vi "Variable Setup GUI.vi"(11 "error in (no error)":errorcluster) -> (8 "OK":bool, 15 "error out":errorcluster)   [LabVIEW 2011]
uses:
  Common/Variable List Common Analog.ctl
  Scaling.ctl
  Action List.ctl
  Alarm Responce.ctl
  Limits.ctl
  Alarm Setup.ctl
  User Setting Analog Channel.ctl
  Update frequensies.ctl
panel:
  out "Sampling Rate":T1
  out "Description":string
  out "Unit":string
  out "Name":string
  in  "User Selectable":T2 {"Limits and responces"."Limits"."H" format="%.3f"; "Limits and responces"."Limits"."L" format="%.3f"; "Limits and responces"."Limits"."HH" format="%.3f"; "Limits and responces"."Limits"."LL" format="%.3f"; "Limits and responces"."HH"."Action" items=["No Action", "Turn Off HV"]; "Limits and responces"."H"."Action" items=["No Action", "Turn Off HV"]; "Limits and responces"."L"."Action" items=["No Action", "Turn Off HV"]; "Limits and responces"."LL"."Action" items=["No Action", "Turn Off HV"]; "Limits and responces"."Technical Error"."Action" items=["No Action", "Turn Off HV"]; "Scaling"."Offset" format="%.5f"; "Scaling"."Gain" format="%.5f"}
  in  "List of variables":i32(listbox)
  out "Mode":bool
  in  "Help":bool
  in  "Cancel":bool
  in  "OK":bool
  # "Information"
  # "Tab header s can be changed as wanted\n\nCustom can be used for completly ccutom behavior,\nmust then highjack  an other hidden page, for settings"
  # "Add custom behavior taht cvan not be replicated by a simple cluster with valisdity checking"
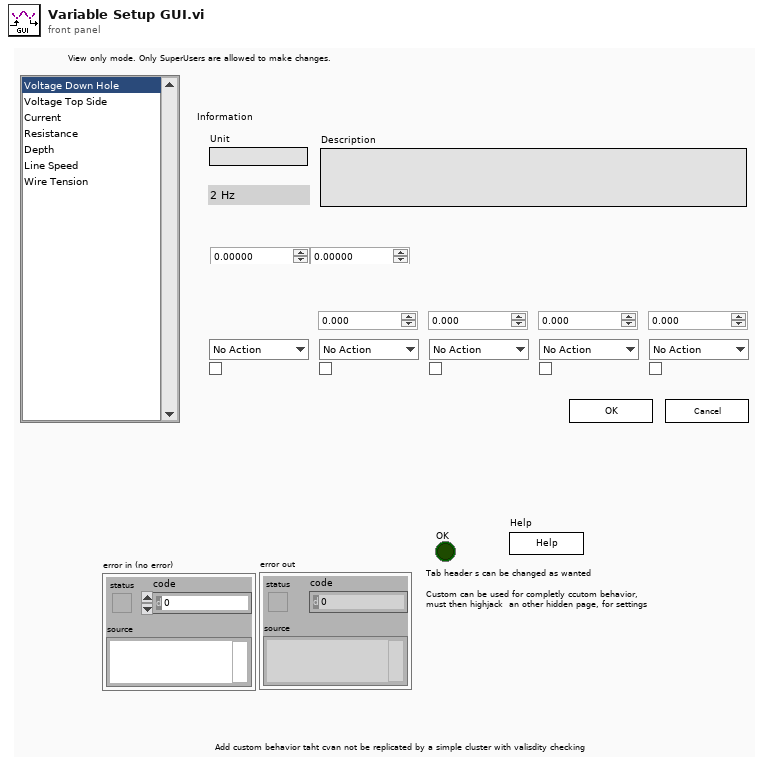
[diagram p1: front panel]
types:
  T1 = typedef "Update frequensies.ctl" = enum16{"2 Hz", "1 Hz", "0.1 Hz"}
  T2 = typedef "User Setting Analog Channel.ctl" = cluster{"Scaling":T3, "Limits and responces":T4}
  T3 = typedef "Scaling.ctl" = cluster{"Gain":dbl, "Offset":dbl}
  T4 = typedef "Alarm Setup.ctl" = cluster{"Technical Error":T5, "LL":T5, "L":T5, "H":T5, "HH":T5, "Limits":T7}
  T5 = typedef "Alarm Responce.ctl" = cluster{"Action":T6, "Alarm":bool}
  T6 = typedef "Action List.ctl" = u16
  T7 = typedef "Limits.ctl" = cluster{"LL":dbl, "L":dbl, "H":dbl, "HH":dbl}
  T8 = enum16{"GET", "SET", "Get from Ini", "Put in Ini"}
  T9 = typedef "User Indikator.ctl" = cluster{"User Name":string, "Super User":T10}
  T10 = typedef "Super User bool indikator.ctl" = bool
  T11 = typedef "Variable List Common Analog.ctl" = enum16{"HVPSU Head Voltage", "HVPSU TS Voltage", "HVPSU Current", "PCP Cable Resistance", "Winch Depth", "Winch Line Speed", "Winch Wire Tension"}
  T12 = enum8{"Enabled", "Disabled", "Disabled and Grayed Out"}
  T13 = typedef "User Setting Analog Channel Bg.ctl" = cluster{"Scaling":T3, "Limits and responces":T14, "Allow Graph selection by user":bool, "Unit":u16}
  T14 = typedef "Alarm Setup Analog.ctl" = cluster{"Technical Error(NA)":T5, "LL":T5, "L":T5, "H":T5, "HH":T5, "Limits":T7}
  T15 = typedef "Fixed Analog Channel Definition.ctl" = cluster{"ID":u16, "Name":string, "Quantity":T16, "Unit":string, "Maximum upd":T1, "Comment":string, "Help file Name":string, "Help file Section ":string, "Category":T17, "User adjustable Scaling":bool, "Default Scaling":T3, "In use":bool, "Default Unit":i32}
  T16 = typedef "Quantity enum.ctl" = enum16{"Acceleration", "Angle", "Current", "Force", "Distance", "Pressure", "Resistance", "Rotational Speed", "Speed", "Temperature", "Tension", "Torque", "Voltage", "Weight"}
  T17 = typedef "Channel catagory Enum.ctl" = enum16{"No Category", "Power", "Temperature", "Pressure"}
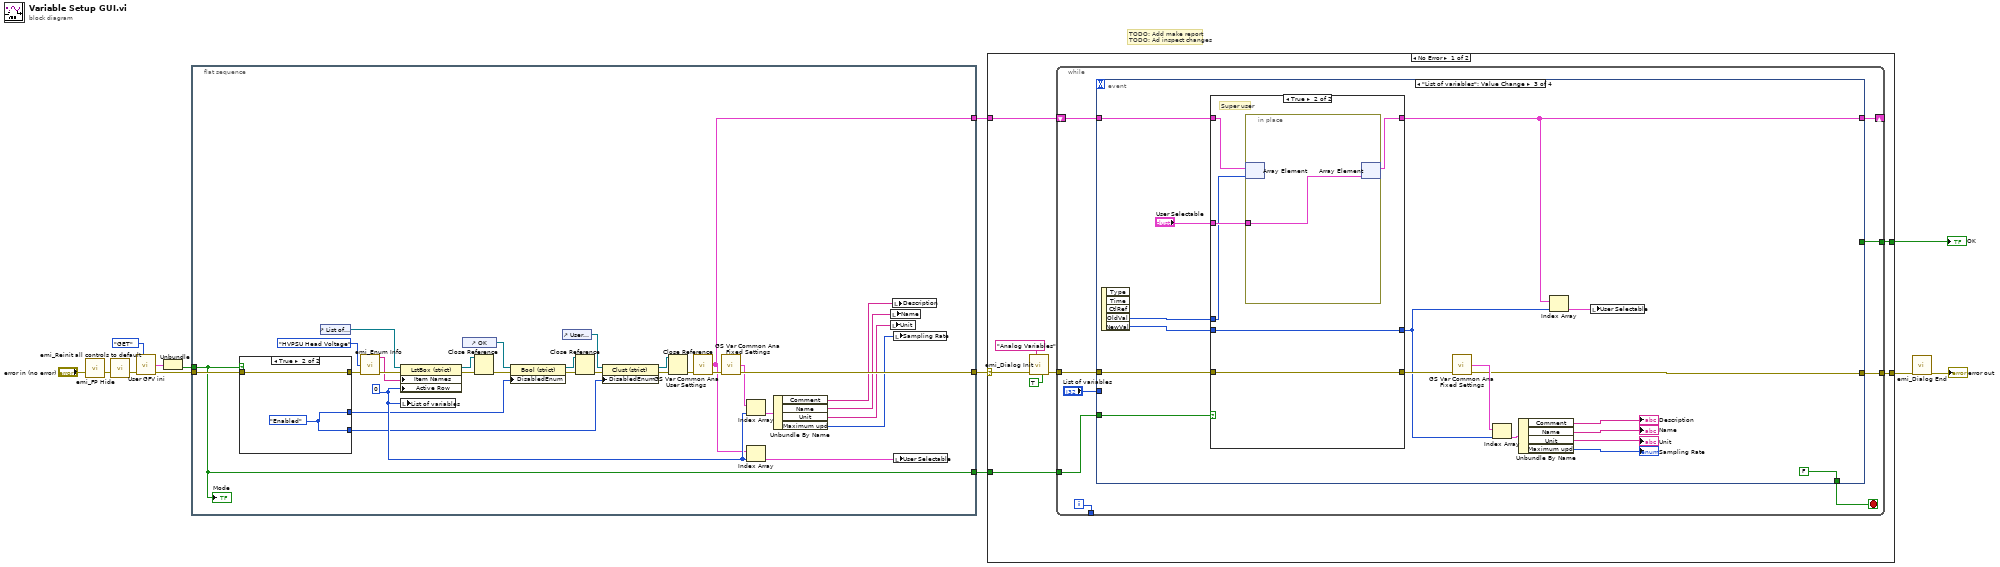
[diagram p0: block diagram]
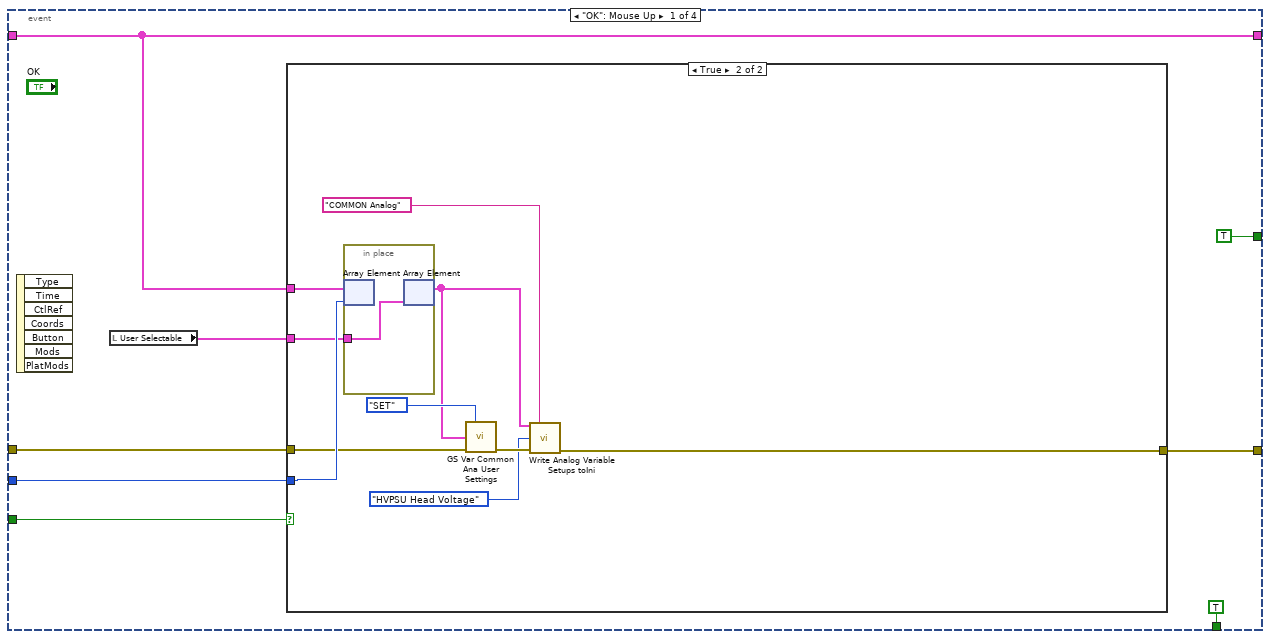
[diagram p2: hidden frame]
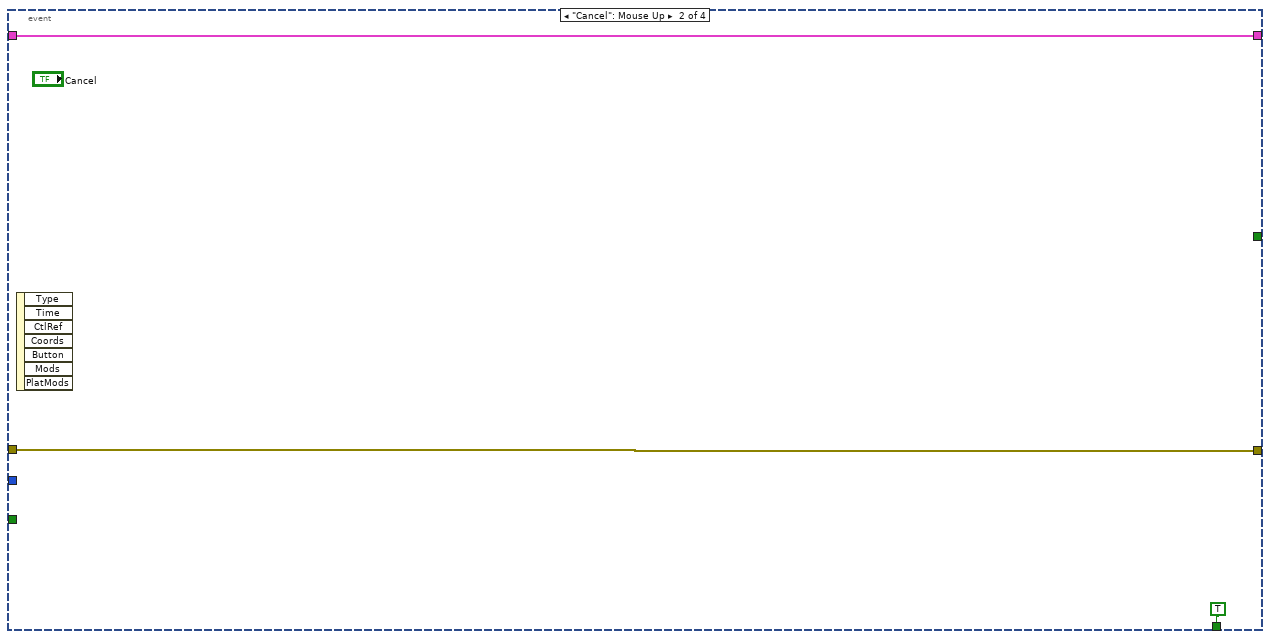
[diagram p4: hidden frame]
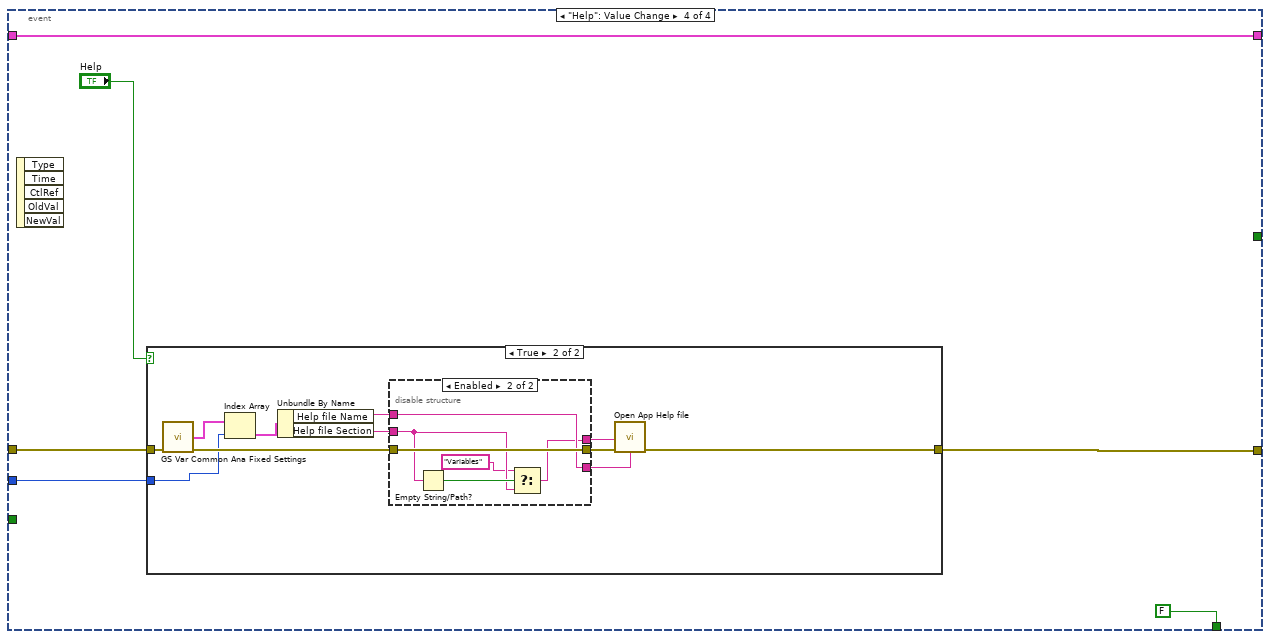
[diagram p6: hidden frame]
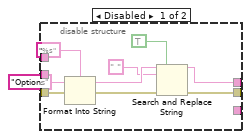
[diagram p8: hidden frame]
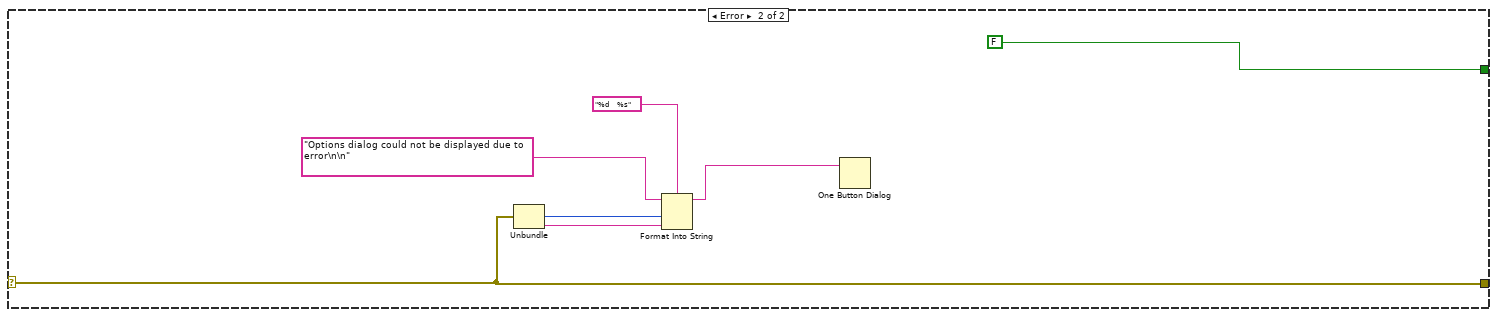
[diagram p9: hidden frame]
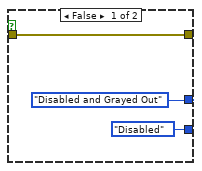
[diagram p10: hidden frame]
diagram:
  # "TODO: Add make report\nTODO: Ad inspect changes"
  n1 = call "emi_FP Hide.vi"("error in (no error)"="error in (no error)") -> ("error out"=w9:errorcluster)  [unwired: 13 in, 1 out]
  n2 = call "emi_Reinit all controls to default.vi"("error in (no error)"=w9) -> ("error out"=w7:errorcluster)  [unwired: 13 in, 1 out]
  n3 = call "User GFV ini.vi"("Action(GET)"=T8."GET", "error in (no error)"=w7) -> ("User ID out"=w6:T9, "error out"=w5:errorcluster)  [unwired: 12 in]
  n4 = Unbundle(w6) -> ("Super User"=w4:T10)  [unwired: 1 out]
  n5 = flat-sequence {
    tunnel: [w31] -> w8
    tunnel: w5 -> [w44]
    tunnel: w4 -> [w17]
    tunnel: [w17] -> w3
    tunnel: [w16] -> w2
    frame #0 {
      w30 = 0 ("Active Row:Active Row Number")
      n6 = case shown="True" w17 {
        tunnel: w44 -> [w46 w49]
        tunnel: [w46 w49] -> w40
        tunnel: [T12."Disabled and Grayed Out" ("Disabled") w48] -> w14
        tunnel: [T12."Disabled" ("Disabled") w48] -> w15
        frame False {
        }
        frame True {
          w48 = T12."Enabled" ("Disabled")
        }
      }
      n7 = control-ref of="List of variables"() -> (w37:refnum<vi>)
      n8 = call "emi_Enum Info.vi"("Enum"=Variable_List_Common_Analog."HVPSU Head Voltage" ("Action"), "error in (no error)"=w40) -> ("Text Elements"=w33:string[], "error out"=w38:errorcluster)  [unwired: 10 in, 2 out]
      n9 = property class="LstBox (strict)"(reference=w37, error in=w38, "Item Names"=w33, "Active Row"=w30) -> (reference out=w35:refnum<vi>, error out=w36:errorcluster)
      n10 = local write "List of variables"(w30) -> ()
      n11 = control-ref of="OK"() -> (w43:refnum<vi>)
      n12 = Close Reference(reference=w35, error in (no error)=w36) -> (error out=w34:errorcluster)
      n13 = property class="Bool (strict)"(reference=w43, error in=w34, "DisabledEnum"=w14) -> (reference out=w41:refnum<vi>, error out=w42:errorcluster)
      n14 = control-ref of="User Selectable"() -> (w18:refnum<vi>)
      n15 = Close Reference(reference=w41, error in (no error)=w42) -> (error out=w19:errorcluster)
      n16 = property class="Clust (strict)"(reference=w18, error in=w19, "DisabledEnum"=w15) -> (reference out=w22:refnum<vi>, error out=w21:errorcluster)
      n17 = Close Reference(reference=w22, error in (no error)=w21) -> (error out=w20:errorcluster)
      n18 = call "GS Var Common Ana User Settings.vi"("error in (no error)"=w20) -> ("Common Analog var User set out"=w16:T13[], "error out"=w32:errorcluster)  [unwired: 12 in, 1 out]
      n19 = call "GS Var Common Ana Fixed Settings.vi"("error in (no error)"=w32) -> ("Common Analog Var Fixed out"=w29:T15[], "error out"=w31:errorcluster)  [unwired: 12 in, 1 out]
      n20 = Index Array(array=w29, index=w30) -> (element=w28:T15)
      n21 = Index Array(array=w16, index=w30) -> (element=w23:T13)
      n22 = Unbundle By Name(w28) -> ("Comment"=w24:string, "Name"=w25:string, "Unit"=w26:string, "Maximum upd"=w27:T1)
      n23 = local write "Unit"(w26) -> ()
      n24 = local write "Name"(w25) -> ()
      n25 = local write "Description"(w24) -> ()
      n26 = local write "Sampling Rate"(w27) -> ()
      n27 = local write "User Selectable"(w23) -> ()
      "Mode" <- w17
    }
  }
  n28 = case shown="No Error" w8 {
    selector: w8 -> [w52 w156]
    tunnel: [w57 FALSE] -> w12
    tunnel: [w56 w156] -> w11
    tunnel: w3 -> [w51 _]
    tunnel: w2 -> [w50 _]
    frame No Error {
      n29 = call "emi_Dialog Init.vi"("Header String(\"\")"="Analog Variables" ("Header String(\"\")"), "error in"=w52, "Modal(T)"=TRUE) -> ("error out"=w55:errorcluster)  [unwired: 12 in]
      n30 = while {
        tunnel: [w66] -> _
        tunnel: w55 -> [w64]
        tunnel: [w63] -> w56
        tunnel: [w62] -> w57
        tunnel: w51 -> [w61]
        shift-right: [w59] -> _
        shift-left: w50 -> [w60]
        i -> [w66]
        stop <- w65 stop-if-true
        n31 = event shown="[2] \"List of variables\": Value Change" {
          selector: _ -> [_ _ _ _]
          dyn-events: _ -> [_ _ _ _]
          timeout: _ -> [_ _ _ _]
          tunnel: [TRUE TRUE FALSE FALSE] -> w65
          tunnel: w64 -> [w73 w88 w105 w121]
          tunnel: [w72 w88 w98 w122] -> w63
          tunnel: [TRUE _ _ _] -> w62
          tunnel: w61 -> [w71 _ w106 _]
          tunnel: w60 -> [w70 w87 w104 w119]
          tunnel: [w70 w87 w92 w119] -> w59
          tunnel: "List of variables" -> [w69 _ _ w118]
          event "OK": Mouse Up {
            n32 = event-data() -> ()  [unwired: 1 in, 7 out]
            n33 = local read "User Selectable"() -> (w68:T2)
            n34 = case shown="True" w71 {
              tunnel: w73 -> [w75 w82]
              tunnel: [w75 w77] -> w72
              tunnel: w70 -> [_ w85]
              tunnel: w69 -> [_ w84]
              tunnel: w68 -> [_ w83]
              frame False {
              }
              frame True {
                n35 = in-place {
                  in-place-border: w83 -> [w86]
                  n36 = in-place-array #1(w85, w84) -> ()  [unwired: 1 out]
                  n37 = in-place-array #1(w86) -> (w78:T13[])  [unwired: 1 out]
                }
                n38 = call "GS Var Common Ana User Settings.vi"("Action(GET)"=enum16{"GET", "SET"}."SET", "Common variables User settigns in"=w78, "error in (no error)"=w82) -> ("error out"=w80:errorcluster)  [unwired: 10 in, 2 out]
                n39 = call "Write Analog Variable Setups toIni.vi"("error in (no error)"=w80, "Enum with Variable List"=Variable_List_Common_Analog."HVPSU Head Voltage" ("Action"), "Analog User settigns"=w78, "Section(\"Default\")"="COMMON Analog" ("Section(\"Default\")")) -> ("error out"=w77:errorcluster)  [unwired: 11 in]
              }
            }
          }
          event "Cancel": Mouse Up {
            n40 = event-data() -> ()  [unwired: 1 in, 7 out]
          }
          event "List of variables": Value Change {
            n41 = event-data() -> ("OldVal"=w103:i32, "NewVal"=w102:i32)  [unwired: 1 in, 3 out]
            n42 = case shown="True" w106 {
              tunnel: [w108 w116] -> w99
              tunnel: w105 -> [w108 w116]
              tunnel: w104 -> [w110 w115]
              tunnel: [w110 w114] -> w92
              tunnel: "User Selectable" -> [_ w113]
              tunnel: w103 -> [_ w112]
              tunnel: w102 -> [w109 w111]
              tunnel: [w109 w111] -> w91
              frame False {
              }
              frame True {
                # "Super user"
                n43 = in-place {
                  in-place-border: w113 -> [w117]
                  n44 = in-place-array #2(w115, w112) -> ()  [unwired: 1 out]
                  n45 = in-place-array #2(w117) -> (w114:T13[])  [unwired: 1 out]
                }
              }
            }
            n46 = call "GS Var Common Ana Fixed Settings.vi"("error in (no error)"=w99) -> ("Common Analog Var Fixed out"=w101:T15[], "error out"=w98:errorcluster)  [unwired: 12 in, 1 out]
            n47 = Index Array(array=w101, index=w91) -> (element=w100:T15)
            n48 = Unbundle By Name(w100) -> ("Comment"=→"Description":string, "Name"=→"Name":string, "Unit"=→"Unit":string, "Maximum upd"=→"Sampling Rate":T1)
            n49 = Index Array(array=w92, index=w91) -> (element=w90:T13)
            n50 = local write "User Selectable"(w90) -> ()
          }
          event "Help": Value Change {
            n51 = event-data() -> ()  [unwired: 1 in, 5 out]
            n52 = case shown="True" "Help" {
              tunnel: [w124 w135] -> w122
              tunnel: w121 -> [w124 w132]
              tunnel: w118 -> [_ w125]
              frame False {
              }
              frame True {
                n53 = call "GS Var Common Ana Fixed Settings.vi"("error in (no error)"=w132) -> ("Common Analog Var Fixed out"=w129:T15[], "error out"=w131:errorcluster)  [unwired: 12 in, 1 out]
                n54 = Index Array(array=w129, index=w125) -> (element=w130:T15)
                n55 = Unbundle By Name(w130) -> ("Help file Name"=w127:string, "Help file Section"=w126:string)
                n56 = disable-structure shown="Enabled" {
                  disable-tunnel: w131 -> [w144 w150]
                  disable-tunnel: [w140 w150] -> w134
                  disable-tunnel: [w136 w146] -> w133
                  disable-tunnel: [_ w149] -> w128
                  disable-tunnel: w127 -> [_ w149]
                  disable-tunnel: w126 -> [_ w147]
                  frame Disabled {
                    n57 = Format Into String(format string="%s", initial string="Options", error in=w144) -> (resulting string=w138:string, error out=w141:errorcluster)  [unwired: 1 in]
                    n58 = Search and Replace String(replace all?=TRUE ("replace all? (F)"), input string=w138, search string=" ", error in=w141) -> (result string=w136:string, error out=w140:errorcluster)  [unwired: 4 in, 2 out]
                  }
                  frame Enabled {
                    n59 = Empty String/Path?(string/path=w147) -> (empty?=w148:bool)
                    n60 = Select(t="Variables", s=w148, f=w147) -> (s? t:f=w146:string)
                  }
                }
                n61 = call "Open App Help file.vi"("Help Tag (\"\")"=w133, "error In"=w134, "file name(\"App\".chm)"=w128) -> ("error out"=w135:errorcluster)  [unwired: 12 in]
              }
            }
          }
        }
      }
    }
    frame Error {
      n62 = Unbundle(w156) -> ("code"=w153:i32, "source"=w152:string)  [unwired: 1 out]
      n63 = Format Into String(format string="%d    %s", initial string="Options dialog could not be displayed due to error\n\n" ("message"), w153, w152) -> (resulting string=w154:string)  [unwired: 1 in, 1 out]
      n64 = One Button Dialog(message=w154) -> ()  [unwired: 1 in, 1 out]
    }
  }
  "OK" <- w12
  n65 = call "emi_Dialog End.vi"("error in"=w11) -> ("error out"=→"error out":errorcluster)  [unwired: 14 in]
